vi "Read Alias.vi"(8 "error in (no error)":errorcluster, 11 "Digital Multimeter in":refnum<class "Digital Multimeter.lvclass">) -> (0 "error out":errorcluster, 2 "Alias":string, 3 "Digital Multimeter out":refnum<class "Digital Multimeter.lvclass">)   [LabVIEW 2020, in "Digital Multimeter.lvclass"]
uses:
  Digital Multimeter.lvclass
  Digital Multimeter.lvclass/Digital Multimeter.ctl
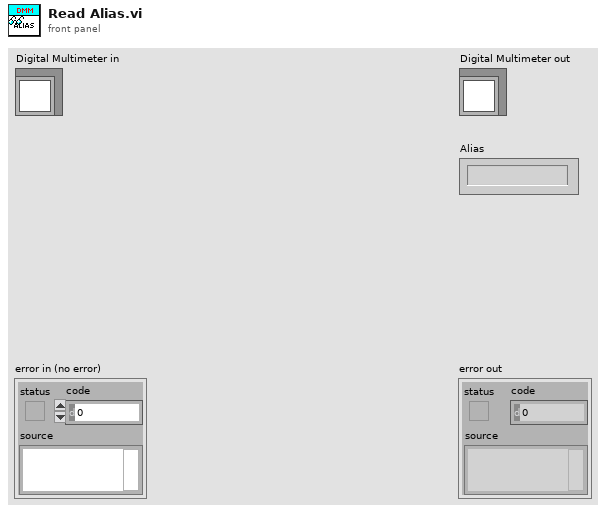
[diagram p1: front panel]
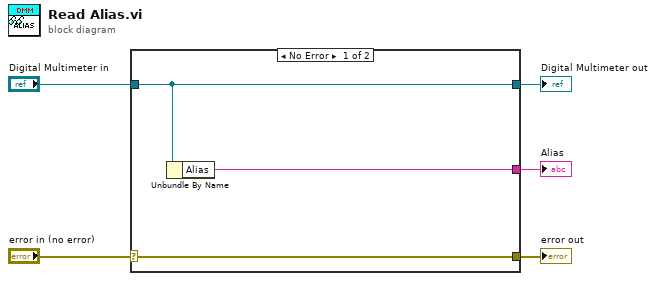
[diagram p0: block diagram]
diagram:
  n1 = case shown="No Error" "error in (no error)" {
    selector: "error in (no error)" -> [w8 w9]
    tunnel: [w8 w9] -> w4
    tunnel: [w7 w10] -> w2
    tunnel: "Digital Multimeter in" -> [w7 w10]
    tunnel: [w6 _] -> w1
    frame No Error {
      n2 = Unbundle By Name(w7) -> ("Alias"=w6:string)
    }
    frame Error {
    }
  }
  "error out" <- w4
  "Digital Multimeter out" <- w2
  "Alias" <- w1
